vi "Init Hardware.vi"(8 "error in (no error)":errorcluster, 11 "ZI Lockin in":refnum<class "ZI Lockin.lvclass">) -> (0 "error out":errorcluster, 3 "ZI Lockin out":refnum<class "ZI Lockin.lvclass">)   [LabVIEW 2018, in "ZI Lockin.lvclass"]
uses:
  ZI Lockin.lvclass
  ZI Lockin.lvclass/ZI Lockin.ctl
  <instrlib>/Zurich Instruments LabOne/Public/ziTypeHandle.ctl
  Read Address.vi
  Write ZI Handle.vi
  <instrlib>/Zurich Instruments LabOne/Zurich Instruments LabOne.lvlib
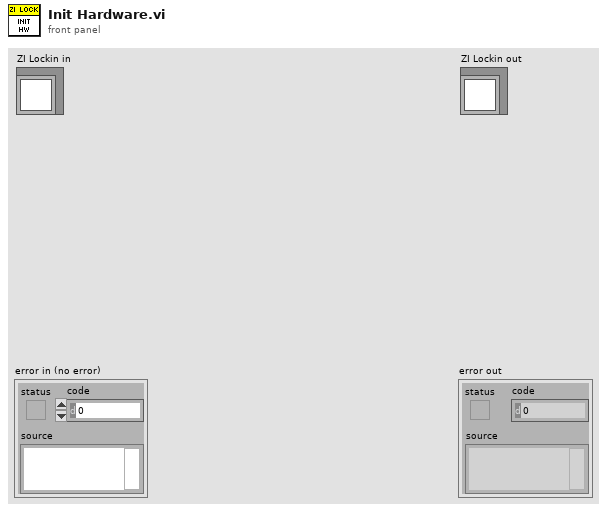
[diagram p1: front panel]
types:
  T1 = typedef "Zurich Instruments LabOne.lvlib/ziTypeHandle.ctl" = cluster{"handleValid":bool, "Conn":u64, "Path Prefix":string, "Handle":u64, "Connected":bool, "Clockbase(s)":dbl}
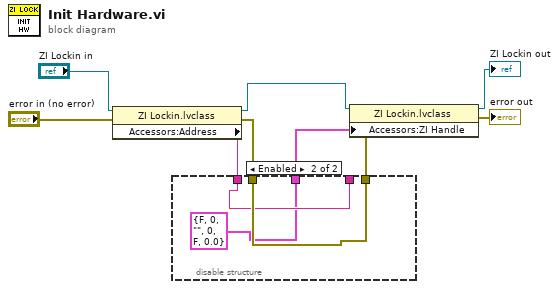
[diagram p0: block diagram]
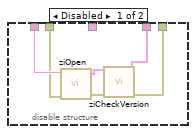
[diagram p2: hidden frame]
diagram:
  n1 = property class="ZI Lockin.lvclass"(reference="ZI Lockin in", error in="error in (no error)") -> (reference out=w6:refnum<class "ZI Lockin.lvclass">, error out=w3:errorcluster, "Accessors:Address"=w7:string)
  n2 = disable-structure shown="Enabled" {
    disable-tunnel: w7 -> [w15 w17]
    disable-tunnel: w3 -> [w14 w18]
    disable-tunnel: [w11 w18] -> w2
    disable-tunnel: [w10 w17] -> _
    disable-tunnel: [_ T1 {"handleValid"=FALSE, "Conn"=0, "Path Prefix"="", "Handle"=0, "Connected"=FALSE, "Clockbase(s)"=0.0} ("ZI Handle")] -> w1
    frame Disabled {
      n3 = call <instrlib>:"ziOpen.vi"("Error In"=w14, "Address"=w15) -> ("Error Out"=w12:errorcluster, "HandleOut"=w13:T1)  [unwired: 2 in, 1 out]
      n4 = call <instrlib>:"ziCheckVersion.vi"("Handle In"=w13, "Error In"=w12) -> ("Handle Out"=w10:T1, "Error Out"=w11:errorcluster)  [unwired: 11 in, 1 out]
    }
    frame Enabled {
    }
  }
  n5 = property class="ZI Lockin.lvclass"(reference=w6, error in=w2, "Accessors:ZI Handle"=w1) -> (reference out=→"ZI Lockin out":refnum<class "ZI Lockin.lvclass">, error out=→"error out":errorcluster)
